vi "Get Data.vi"(8 "error in (no error)":errorcluster, 10 "Bus In":refnum<class "Bus.lvclass">, 11 "No Query in":refnum<class "No Query.lvclass">) -> (0 "error out":errorcluster, 1 "String Read":string, 2 "Bus Out":refnum<class "Bus.lvclass">, 3 "No Query out":refnum<class "No Query.lvclass">)   [LabVIEW 2015, in "No Query.lvclass"]
doc: "Query.lvclass:Get Data.vi\n\nThis is the template for the Get Data VI for the Query class.\n\nInstrument Communication Module Version 1.0\nSeptember, 2017 Original Code Consulting David Thomson\n www.originalcode.com"
uses:
  No Query.lvclass
  Bus/Bus.lvclass
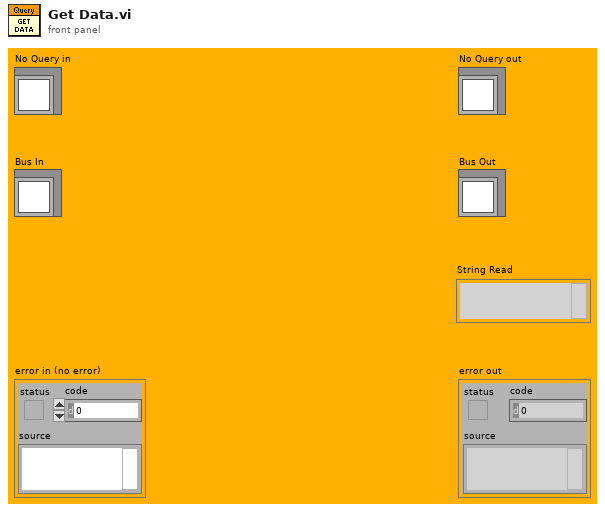
[diagram p1: front panel]
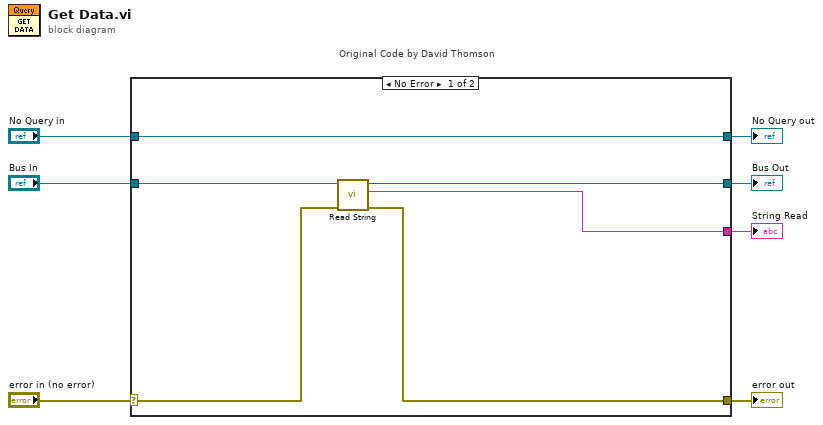
[diagram p0: block diagram]
diagram:
  n1 = case "Original Code by David Thomson" shown="No Error" "error in (no error)" {
    selector: "error in (no error)" -> [w10 w16]
    tunnel: [w9 w16] -> w6
    tunnel: [w13 w15] -> w4
    tunnel: "No Query in" -> [w13 w15]
    tunnel: [w11 w14] -> w3
    tunnel: "Bus In" -> [w12 w14]
    tunnel: [w8 _] -> w1
    frame No Error {
      n2 = call-dynamic "Read String.vi"("error in (no error)"=w10, "Bus in"=w12) -> ("error out"=w9:errorcluster, "String Read"=w8:string, "Bus out"=w11:refnum<class "Bus.lvclass">)  [unwired: 6 in, 1 out]
    }
    frame Error {
    }
  }
  "error out" <- w6
  "No Query out" <- w4
  "Bus Out" <- w3
  "String Read" <- w1
